vi "modem_reset.vi"(2 "error in (no error)":errorcluster, 3 "VISA resource name":refnum<visa-resource-name>="COM1") -> (0 "error out":errorcluster, 1 "read buffer":string)   [LabVIEW 2010]
uses:
  <vilib>/Instr/_visa.llb/VISA Configure Serial Port (Instr).vi
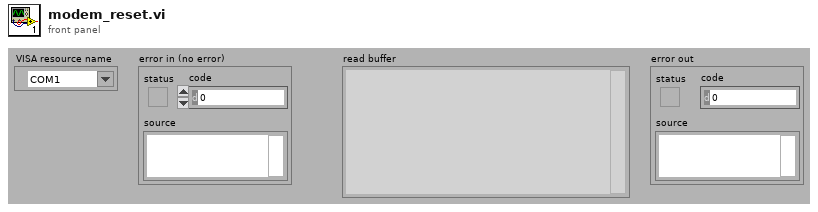
[diagram p1: front panel]
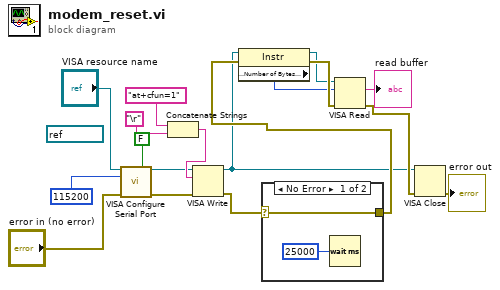
[diagram p0: block diagram]
diagram:
  (unwired) refnum<visa-resource-name> "COM1" ("VISA resource name")
  n1 = call-poly "VISA Configure Serial Port"("VISA resource name"="VISA resource name", "Enable Termination\nChar (T)"=FALSE ("Enable Termination\nChar (T)"), "baud rate (9600)"=u32 115200, "error in (no error)"="error in (no error)") -> ("VISA resource name out"=w4:refnum<visa-resource-name>, "error out"=w3:errorcluster)  [unwired: 10 in]
  n2 = Concatenate Strings("at+cfun=1" ("write buffer"), "\r") -> (w17:string)
  n3 = VISA Write(VISA resource name=w4, write buffer=w17, error in (no error)=w3) -> (VISA resource name out=w8:refnum<visa-resource-name>, error out=w7:errorcluster)  [unwired: 1 out]
  n4 = case shown="No Error" w7 {
    selector: w7 -> [w19 w21]
    tunnel: [w19 w21] -> w12
    frame No Error {
      n5 = Wait (ms)(milliseconds to wait=u32 25000) -> ()  [unwired: 1 out]
    }
    frame Error {
    }
  }
  n6 = property class="Instr"(reference=w8, error in=w12) -> (reference out=w9:refnum<visa-resource-name>, error out=w13:errorcluster, "Serial Settings:Number of Bytes at Serial Port"=w10:u32)
  n7 = VISA Read(VISA resource name=w9, byte count=w10, error in (no error)=w13) -> (read buffer=→"read buffer":string, error out=w14:errorcluster)  [unwired: 2 out]
  n8 = VISA Close(VISA resource name=w8, error in (no error)=w14) -> (error out=→"error out":errorcluster)
